vi "Library File Name to Display Name.vi"(8 "error in (no error)":errorcluster, 11 "Library Name":string) -> (0 "error out":errorcluster, 3 "Display Name":string)   [LabVIEW 2019, in "NIPKG Naming.lvlib"]
uses:
  NIPKG Naming.lvlib
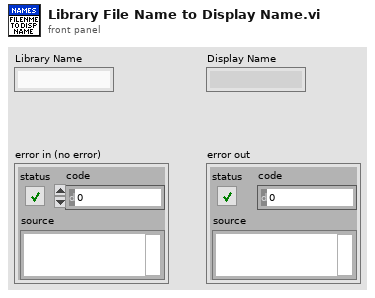
[diagram p1: front panel]
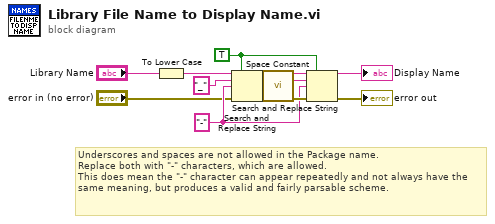
[diagram p0: block diagram]
diagram:
  w7 = TRUE ("replace all? (F)")
  w9 = "-" ("replace string (\"\")")
  # "Underscores and spaces are not allowed in the Package name.\nReplace both with \"-\" characters, which are allowed.\nThis does mean the \"-\" character can appear repeatedly and not always have the same meaning, but produces a valid and fairly parsable scheme."
  n1 = To Lower Case(string="Library Name") -> (all lower case string=w11:string)
  n2 = Search and Replace String(replace all?=w7, input string=w11, search string="_", replace string=w9, error in="error in (no error)") -> (result string=w6:string, error out=w10:errorcluster)  [unwired: 3 in, 2 out]
  n3 = call <vilib>:"Space Constant.vi"() -> ("String"=w8:string)
  n4 = Search and Replace String(replace all?=w7, input string=w6, search string=w8, replace string=w9, error in=w10) -> (result string=→"Display Name":string, error out=→"error out":errorcluster)  [unwired: 3 in, 2 out]
